vi "Material-ProcessResults.vi"(8 "error in (no error)":errorcluster, 11 "Material-RunTest in":refnum<class "Material-RunTest.lvclass">) -> (0 "error out":errorcluster, 3 "Material-RunTest out":refnum<class "Material-RunTest.lvclass">)   [LabVIEW 2013, in "Material-RunTest.lvclass"]
uses:
  Material-RunTest.lvclass
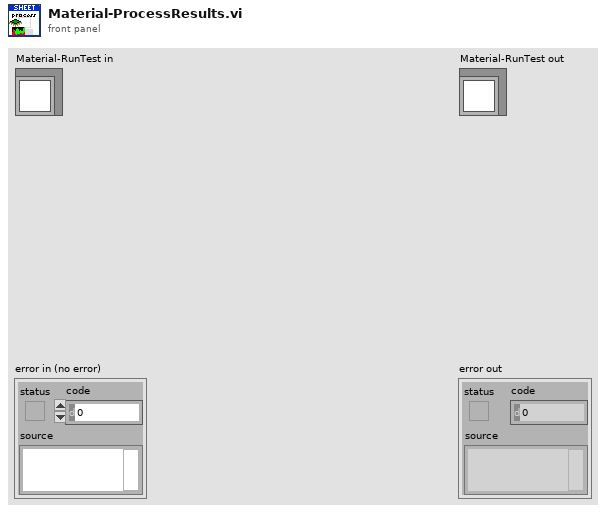
[diagram p1: front panel]
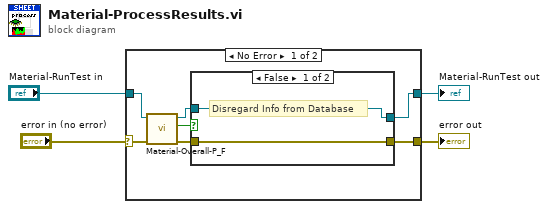
[diagram p0: block diagram]
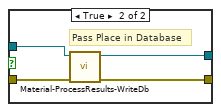
[diagram p2: hidden frame]
diagram:
  n1 = case shown="No Error" "error in (no error)" {
    selector: "error in (no error)" -> [w10 w19]
    tunnel: [w5 w19] -> w3
    tunnel: [w6 w18] -> w1
    tunnel: "Material-RunTest in" -> [w11 w18]
    frame No Error {
      n2 = call "Material-Overall-P_F.vi"("error in"=w10, "Material-RunTest in"=w11) -> ("error out"=w7:errorcluster, "Sheet Overall Passed?"=w9:bool, "Material-RunTest in 2"=w8:refnum<class "Material-RunTest.lvclass">)  [unwired: 7 in]
      n3 = case shown="False" w9 {
        tunnel: w8 -> [w13 w16]
        tunnel: w7 -> [w12 w17]
        tunnel: [w12 w15] -> w5
        tunnel: [w13 w14] -> w6
        frame False {
          # "Disregard Info from Database"
        }
        frame True {
          # "Pass Place in Database"
          n4 = call "Material-ProcessResults-WriteDb.vi"("error in (no error)"=w17, "Material-RunTest in"=w16) -> ("error out"=w15:errorcluster, "Material-RunTest out"=w14:refnum<class "Material-RunTest.lvclass">)  [unwired: 8 in]
        }
      }
    }
    frame Error {
    }
  }
  "error out" <- w3
  "Material-RunTest out" <- w1
